vi "收集数据ICRA2024测试椭圆分裂.vi"() -> ()   [LabVIEW 2018]
doc: "Demonstrates the use of the Network Streams functions to send LED status to the myRIO target."
uses:
  <vilib>/ErrorRing/Error Ring.xnode
  <vilib>/vision/NI_Vision_Development_Module.lvlib
panel:
  out "面积":sgl[](array[numeric])
  out "面积":sgl
  out "数据总":dbl[][](array[numeric])
  out "i":i32[](array[numeric])
  out "aspect ratio":dbl[](array[numeric])
  out "D2":i32[](array[numeric])
  out "D1":i32[](array[numeric])
  out "field ratio":sgl[](array[numeric])
  out "field ratio":sgl=4.0
  out "时间":i32
  in  "打开数据记录":bool
  out "aspect ratio":dbl
  out "D2":i32
  out "D1":i32
  out "二值图":T1(plugin-control)
  in  "Search Rect (entire image)":T2={"Left"=200, "Top"=120, "Right"=2000, "Bottom"=1920, "Rotation"=0.0} {"Rotation" format="%.2f"; "Left" scale=0.0..1024.0; "Right" scale=0.0..1024.0}
  out "备用的椭圆角度":sgl
  in  "Number of Erosion":i32=10
  in  "椭圆磁场开关":bool=TRUE
  out "Image 7":T1(plugin-control)
  in  "Acquisition Control::Acquisition Frame Rate":dbl=19.50304412841797 min=1.4211589097976685 max=44.94382095336914
  out "Stopped":bool
  in  "Stop (F) 2":bool caption="Stop (F)"
  out "Objects 2":T3(array[cluster]) {"Aspect Ratio" format="%.2f"; "Orientation" format="%.2f"; "Area" format="%.2f"; "Object Center"."Y" format="%.2f"; "Object Center"."X" format="%.2f"}
  in  "Settings 2":T4={"Objects"=0, "Threshold"=128, "Reject Border"=FALSE, "Fill Holes"=FALSE, "Min Object Size"=TRUE, "Min Size"=20000, "Max Object Size"=FALSE, "Max Size"=100, "Show Search Area"=FALSE, "Show Center"=TRUE, "Show Bounding Box"=TRUE} {"Objects" items=["Bright Objects", "Dark Objects"]; "Threshold" min=1 max=999999999 step=1; "Max Size" min=1 max=999999999 step=1; "Min Size" min=1 max=999999999 step=1}
  in  "Range 2":cluster{"Lower value":sgl, "Upper value":sgl}={"Lower value"=0.0, "Upper value"=230.0} {"Upper value" format="%.2f"; "Lower value" format="%.2f"}
  in  "Pause":bool
  out "Array":dbl[](array[numeric])
  in  "Parameter Settings":T5(tab)=enum."Ribbon Oscillating Field" caption="Field Types"
  in  "fg":dbl
  in  "pg":dbl
  in  "dg":dbl
  in  "Ag":dbl
  in  "AoOF":dbl
  in  "fo":sgl
  in  "do":sgl
  in  "oo":sgl
  in  "po":sgl
  in  "cc":sgl
  in  "pc":sgl
  in  "wc":sgl
  in  "dc":sgl
  in  "Ac":dbl
  in  "pr":sgl
  in  "Ar":dbl=8.0
  in  "wr":sgl=18.0
  in  "dr":sgl
  in  "Dis phase step":dbl
  in  "Dis phase frequency (Hz)":dbl
  in  "Dis tumbling frequency (Hz)":dbl
  in  "Dis strength(mT)":dbl
  in  "Swa strength (mT)":dbl
  in  "Swa frequency (Hz)":dbl
  in  "Swa pitch angle (deg)":dbl
  in  "Swa direction angle (deg)":dbl
  in  "Swa ratio":dbl=1.0
  in  "Pitch Angle (rotating around Constant, deg)":dbl
  in  "Ratio (A/C)":sgl=4.0
  in  "Direction Angle (deg)":sgl
  in  "Pitch Angle (rotating around Origin, deg)":sgl
  in  "Frequency (Hz)":sgl=10.0
  in  "Strength (mT)":dbl=10.0
  in  "Ar 2":dbl=5.0 caption="Ar"
  in  "ratio":sgl=1.0
  in  "运动方向":sgl
  in  "长轴方向":sgl
  in  "wr  2":sgl=8.0
  in  "速度大小":sgl
  out "Numeric 5":i32
  in  "Stop":bool
  out "error out":errorcluster
  in  "Target IP Address":string="172.22.11.2"
  # "Overview: Magnetic field calculation, and send parameters to myRIO\nInstructions:\n1. Verify the value of Target IP Address. Set Visa resource name.\n2. Ensure RT Main.vi is already running. \n3. Run this VI. Set parameters of magnetic field."
  # "Strength (mT)"
  # "Pitch Angle (deg)"
  # "Direction Angle (deg)"
  # "Frequency (Hz)"
  # "Strength (mT)"
  # "Oscilation Frequency (Hz)"
  # "Oscilation Angle (deg)"
  # "Pitch Angle (deg)"
  # "Direction Angle (deg)"
  # "Strength (mT)"
  # "Frequency (Hz)"
  # "Pitch Angle (deg)"
  # "Direction Angle (deg)"
  # "Conical Angle (deg)"
  # "Strength (mT)"
  # "Frequency (Hz)"
  # "Pitch Angle (deg)"
  # "Direction Angle (deg)"
  # "Strength (mT)"
  # "Tumbling Frequency (Hz)"
  # "Phase Frequency (Hz)"
  # "Phase Step"
  # "Strength (mT)"
  # "Frequency (Hz)"
  # "Pitch Angle (deg)"
  # "Direction Angle (deg)"
  # "Ratio"
  # "Strength (mT)"
  # "Frequency (Hz)"
  # "Ratio (A/C)"
  # "Direction Angle (deg)"
  # "Pitch Angle (rotating around Origin, deg)"
  # "Pitch Angle (rotating around Constant, deg)"
  # "Strength (mT)"
  # "Frequency (Hz)"
  # "Pitch Angle  (deg)"
  # "longaxis"
  # "Direction Angle (deg)"
  # "ratio (l/s)"
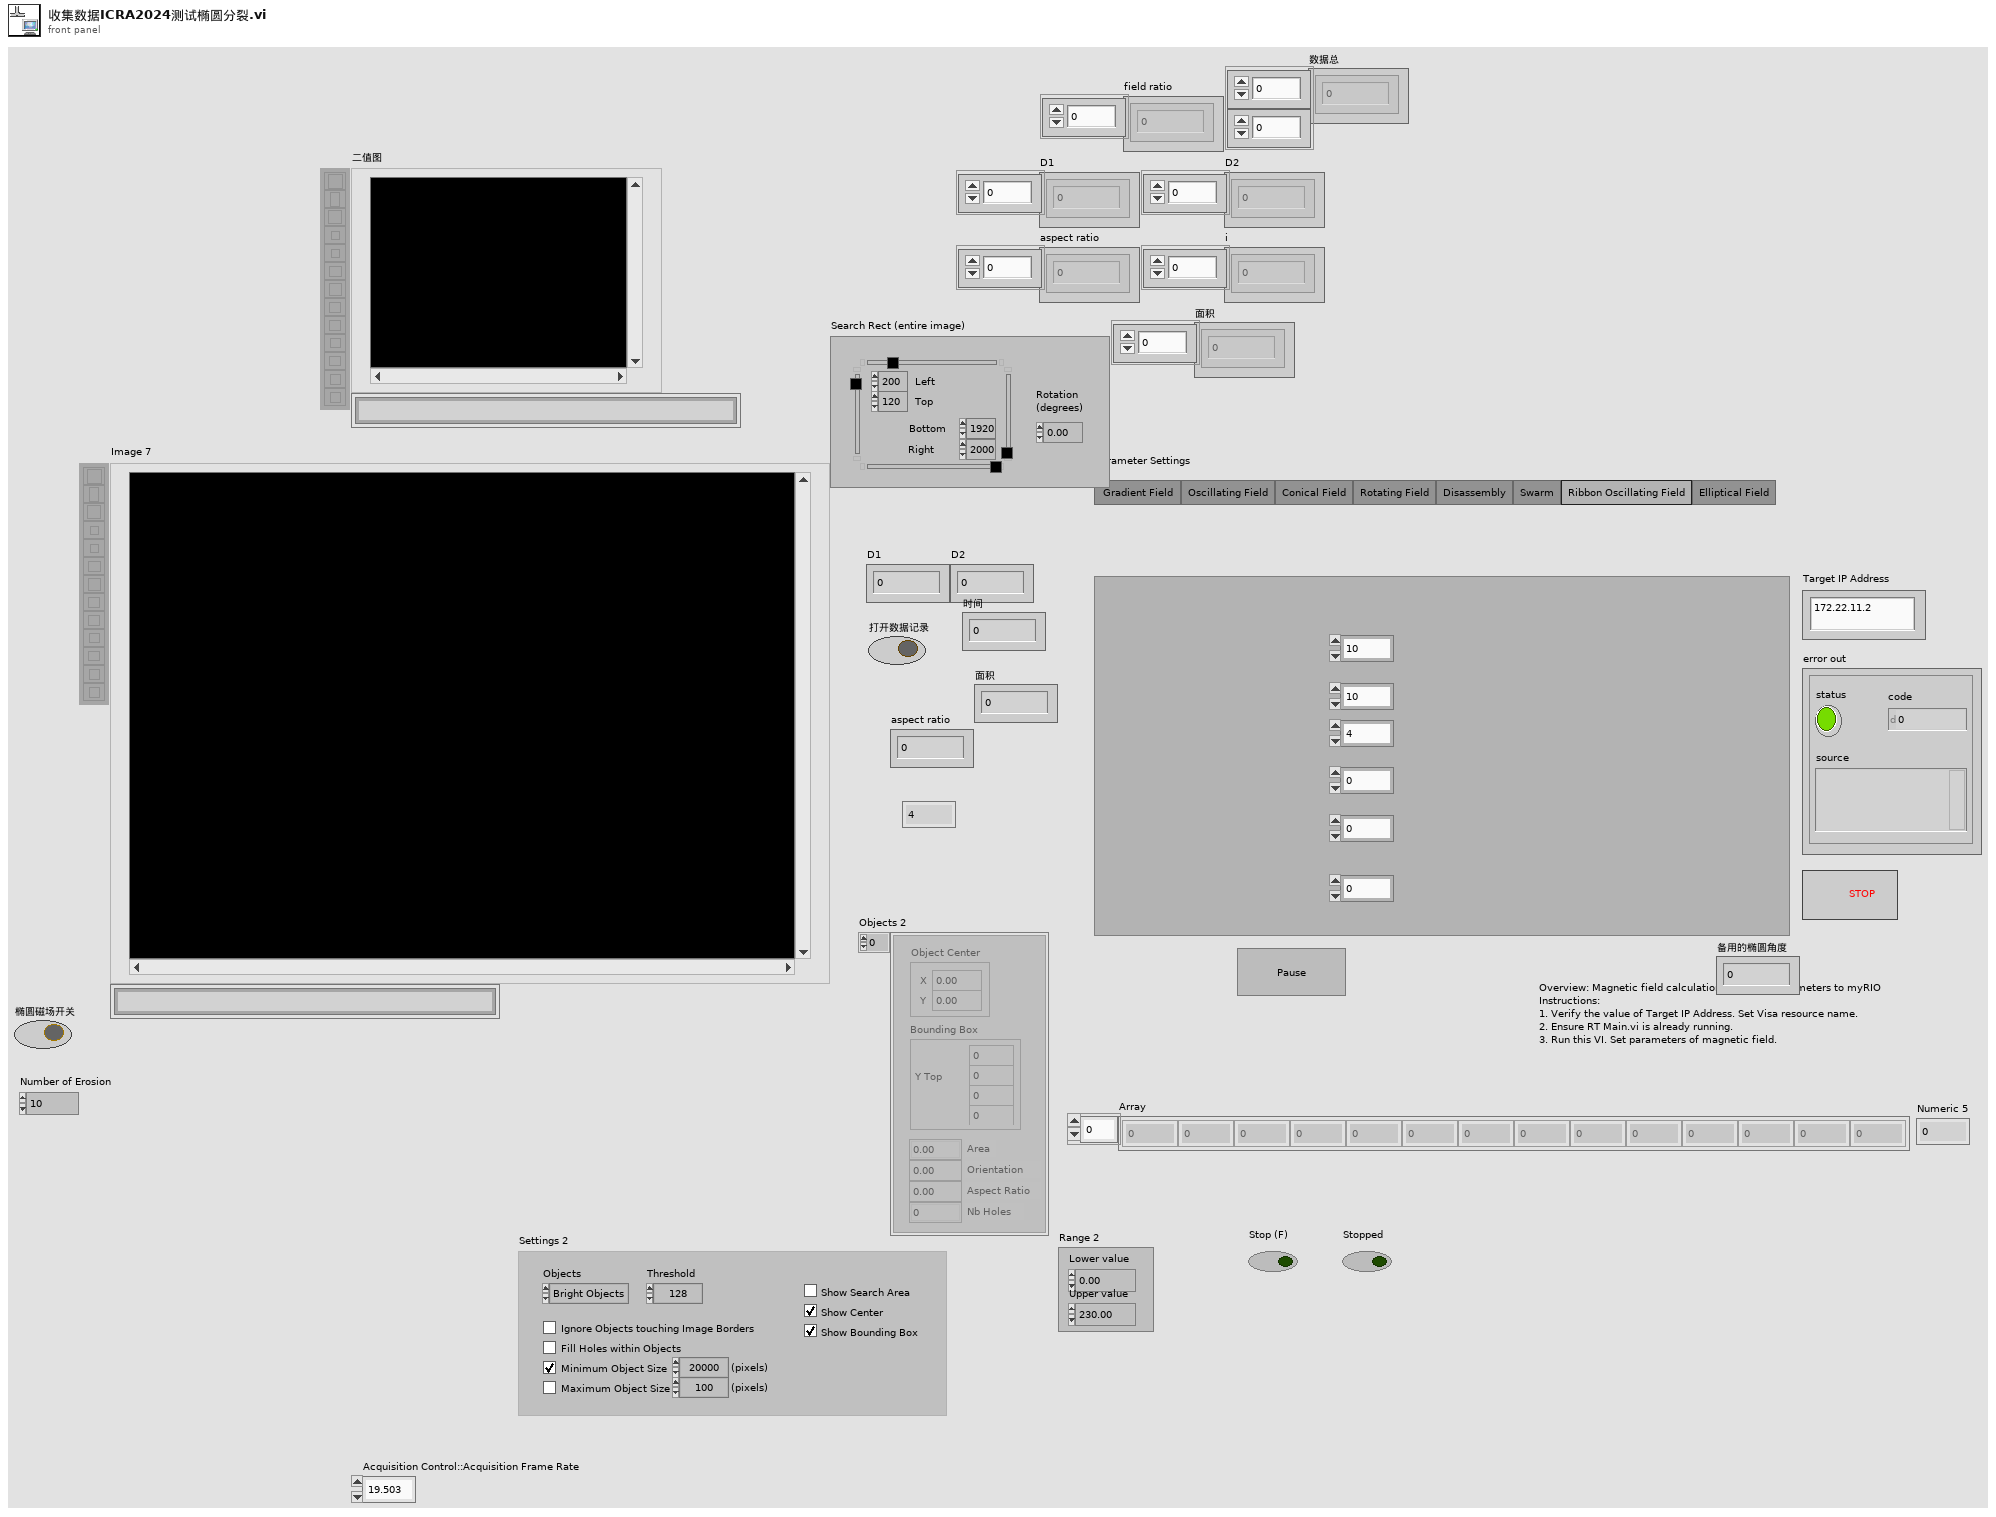
[diagram p1: front panel]
types:
  T1 = typedef "IMAQ Image.ctl" = refnum<image>
  T2 = typedef "IMAQ Rectangle" = cluster{"Left":i32, "Top":i32, "Right":i32, "Bottom":i32, "Rotation":dbl}
  T3 = cluster{"Object Center":cluster{"X":sgl, "Y":sgl}, "Bounding Box":cluster{"X Left":i32, "Y Top":i32, "X Right":i32, "Y Bottom":i32}, "Area":sgl, "Orientation":sgl, "Aspect Ratio":sgl, "Nb Holes":i32}[]
  T4 = cluster{"Objects":u16, "Threshold":i32, "Reject Border":bool, "Fill Holes":bool, "Min Object Size":bool, "Min Size":i32, "Max Object Size":bool, "Max Size":i32, "Show Search Area":bool, "Show Center":bool, "Show Bounding Box":bool}
  T5 = enum32{"Gradient Field ", "Oscillating Field", "Conical Field", "Rotating Field", "Disassembly", "Swarm", "Ribbon Oscillating Field", "Elliptical Field"}
  T6 = typedef "Image Type" = u32
  T7 = cluster{"Objects[0]":cluster{"Object Center":cluster{"X":sgl, "Y":sgl}, "Bounding Box":cluster{"X Left":i32, "Y Top":i32, "X Right":i32, "Y Bottom":i32}, "Area":sgl, "Orientation":sgl, "Aspect Ratio":sgl, "Nb Holes":i32}, "Objects[1]":cluster{"Object Center":cluster{"X":sgl, "Y":sgl}, "Bounding Box":cluster{"X Left":i32, "Y Top":i32, "X Right":i32, "Y Bottom":i32}, "Area":sgl, "Orientation":sgl, "Aspect Ratio":sgl, "Nb Holes":i32}, "Objects[2]":cluster{"Object Center":cluster{"X":sgl, "Y":sgl}, "Bounding Box":cluster{"X Left":i32, "Y Top":i32, "X Right":i32, "Y Bottom":i32}, "Area":sgl, "Orientation":sgl, "Aspect Ratio":sgl, "Nb Holes":i32}, "Objects[3]":cluster{"Object Center":cluster{"X":sgl, "Y":sgl}, "Bounding Box":cluster{"X Left":i32, "Y Top":i32, "X Right":i32, "Y Bottom":i32}, "Area":sgl, "Orientation":sgl, "Aspect Ratio":sgl, "Nb Holes":i32}, "Objects[4]":cluster{"Object Center":cluster{"X":sgl, "Y":sgl}, "Bounding Box":cluster{"X Left":i32, "Y Top":i32, "X Right":i32, "Y Bottom":i32}, "Area":sgl, "Orientation":sgl, "Aspect Ratio":sgl, "Nb Holes":i32}, "Objects[5]":cluster{"Object Center":cluster{"X":sgl, "Y":sgl}, "Bounding Box":cluster{"X Left":i32, "Y Top":i32, "X Right":i32, "Y Bottom":i32}, "Area":sgl, "Orientation":sgl, "Aspect Ratio":sgl, "Nb Holes":i32}, "Objects[6]":cluster{"Object Center":cluster{"X":sgl, "Y":sgl}, "Bounding Box":cluster{"X Left":i32, "Y Top":i32, "X Right":i32, "Y Bottom":i32}, "Area":sgl, "Orientation":sgl, "Aspect Ratio":sgl, "Nb Holes":i32}, "Objects[7]":cluster{"Object Center":cluster{"X":sgl, "Y":sgl}, "Bounding Box":cluster{"X Left":i32, "Y Top":i32, "X Right":i32, "Y Bottom":i32}, "Area":sgl, "Orientation":sgl, "Aspect Ratio":sgl, "Nb Holes":i32}, "Objects[8]":cluster{"Object Center":cluster{"X":sgl, "Y":sgl}, "Bounding Box":cluster{"X Left":i32, "Y Top":i32, "X Right":i32, "Y Bottom":i32}, "Area":sgl, "Orientation":sgl, "Aspect Ratio":sgl, "Nb Holes":i32}}
  T8 = cluster{"Object Center":cluster{"X":sgl, "Y":sgl}, "Bounding Box":cluster{"X Left":i32, "Y Top":i32, "X Right":i32, "Y Bottom":i32}, "Area":sgl, "Orientation":sgl, "Aspect Ratio":sgl, "Nb Holes":i32}
  T9 = cluster{"X Left":i32, "Y Top":i32, "X Right":i32, "Y Bottom":i32}
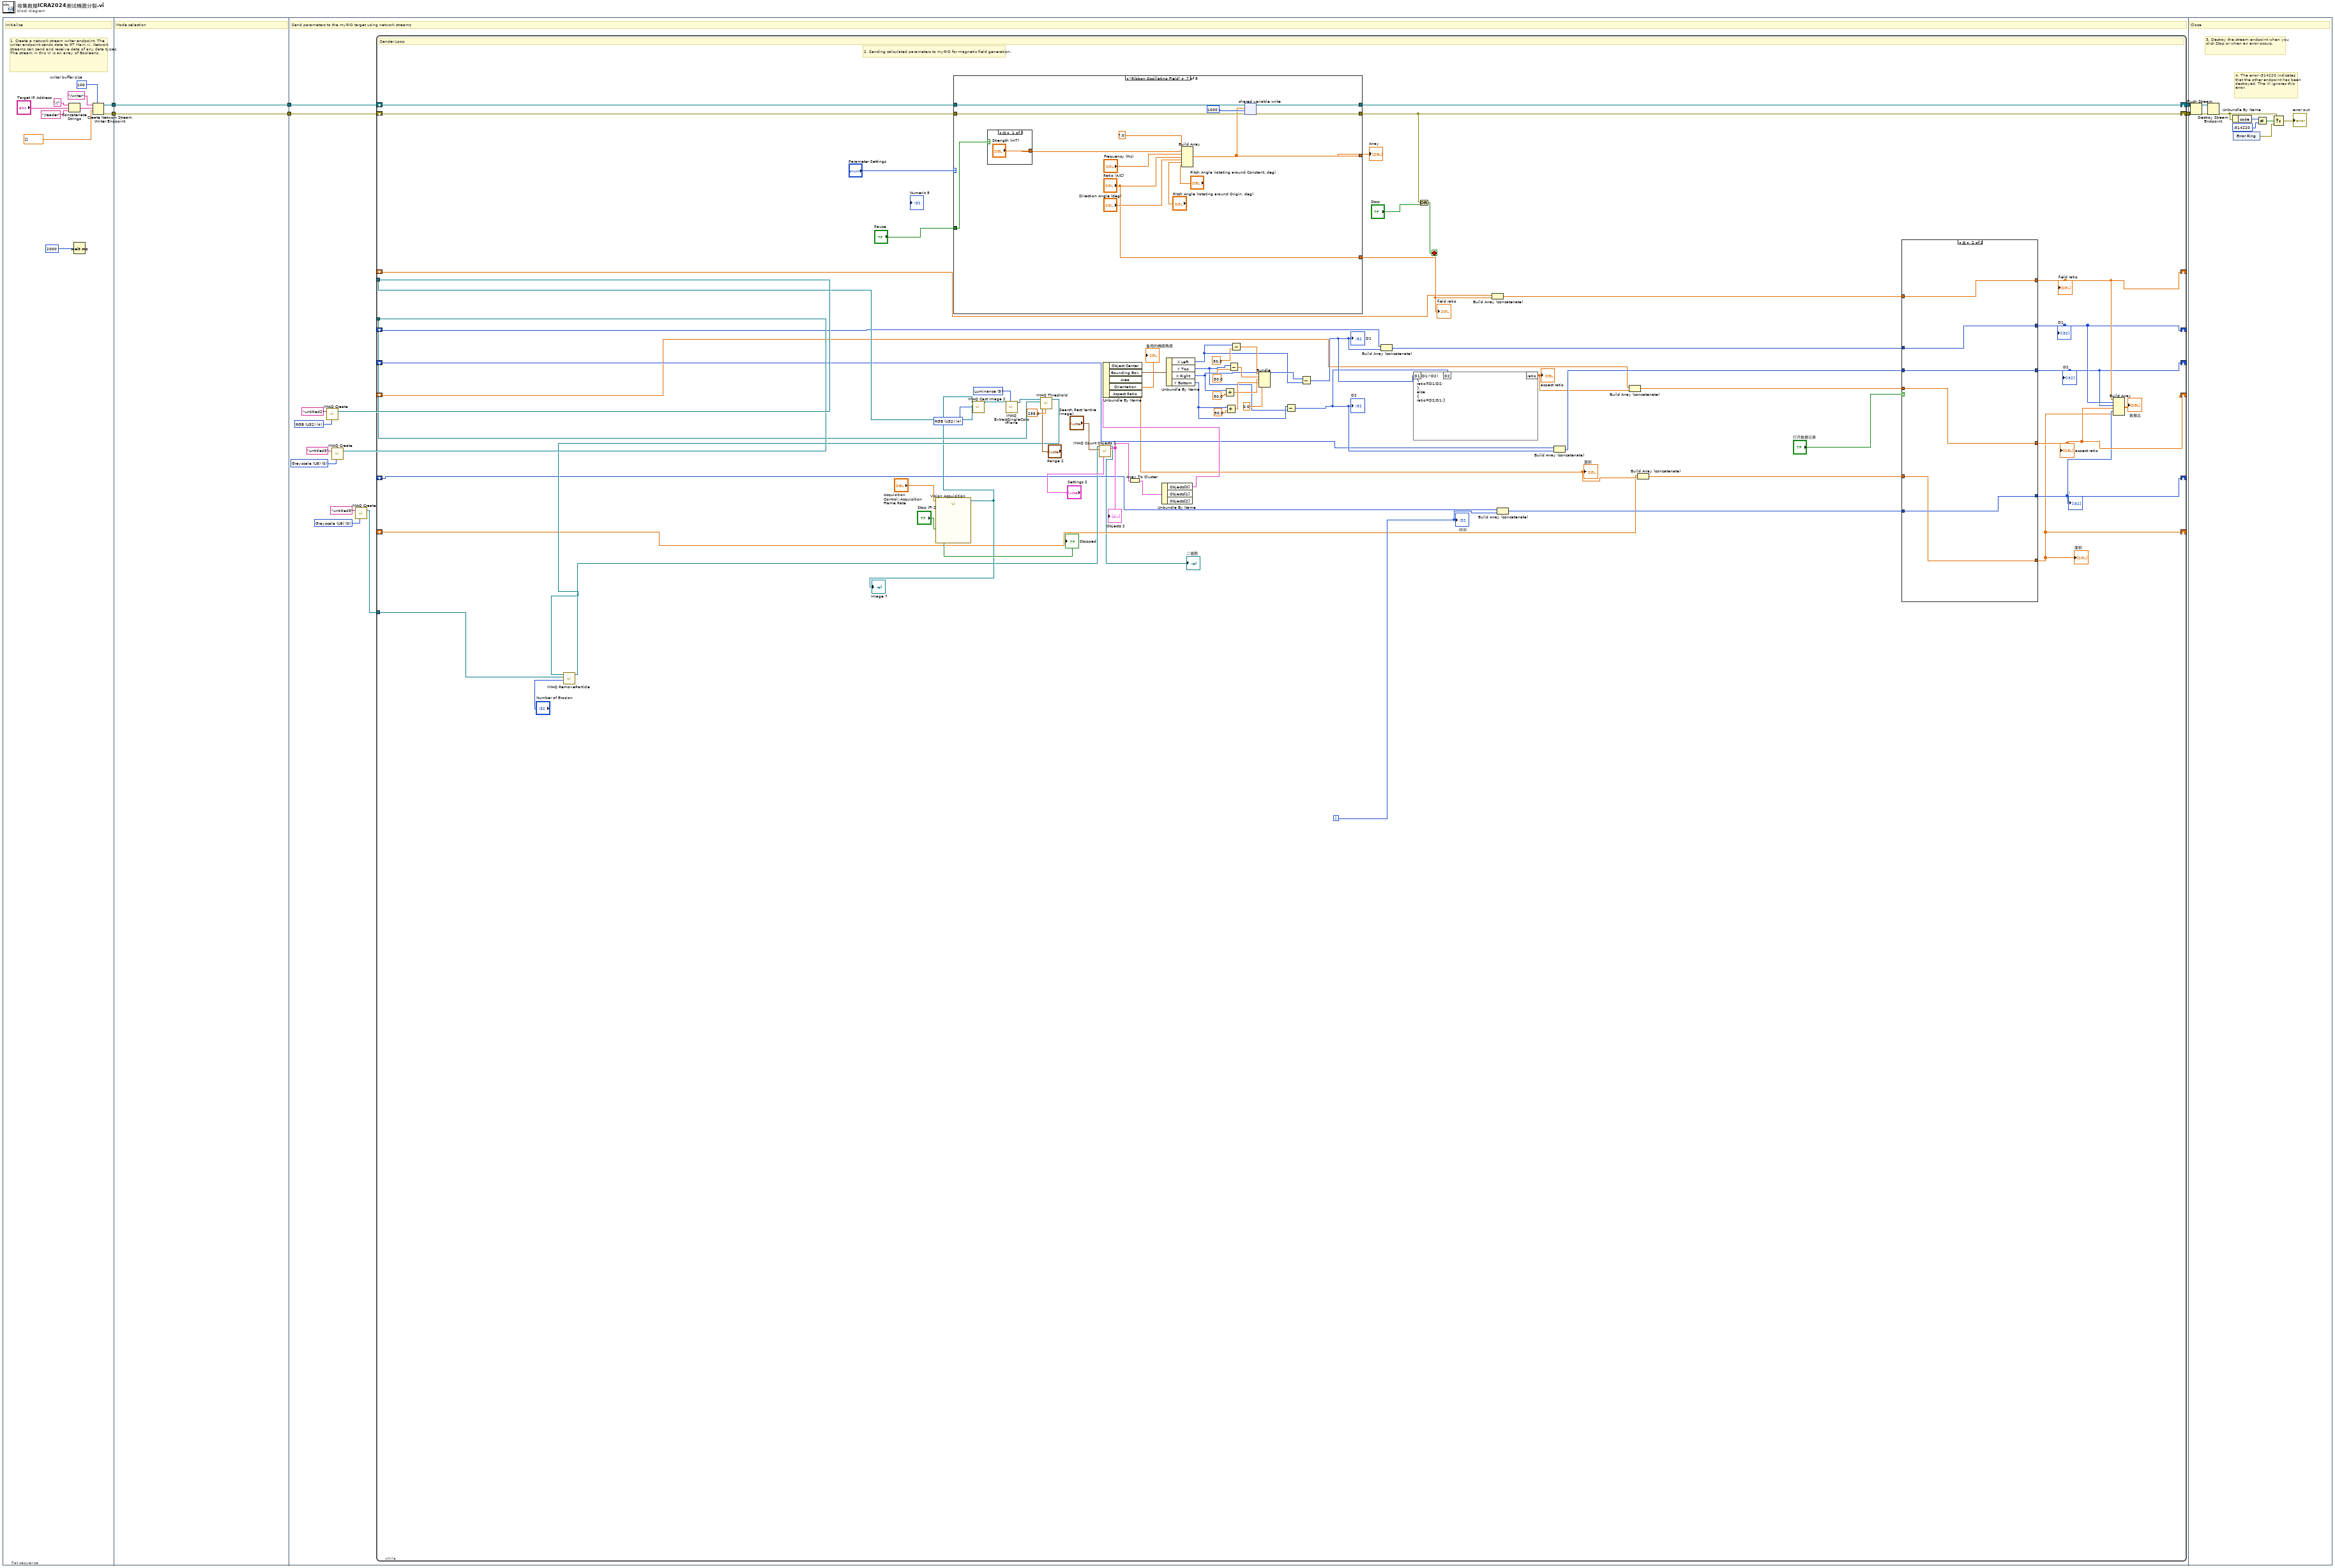
[diagram p0: block diagram]
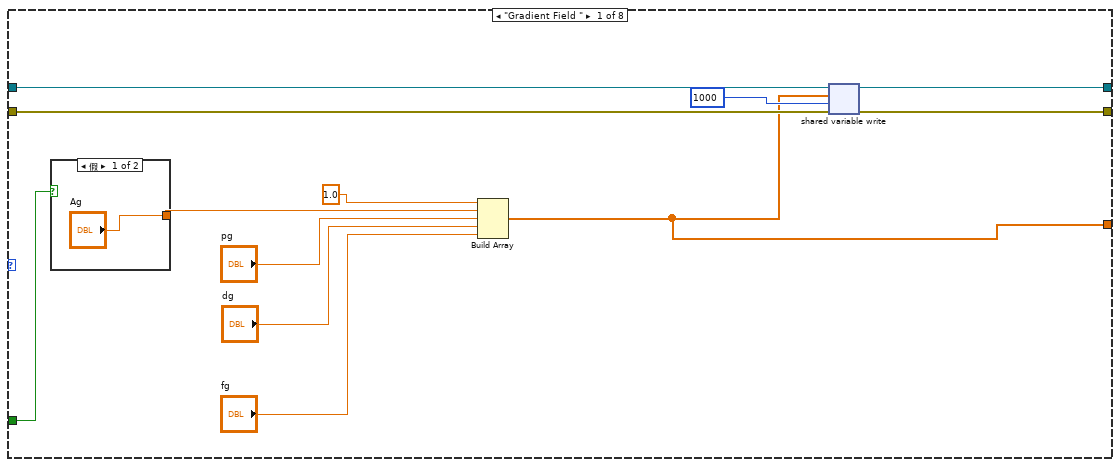
[diagram p3: hidden frame]
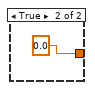
[diagram p4: hidden frame]
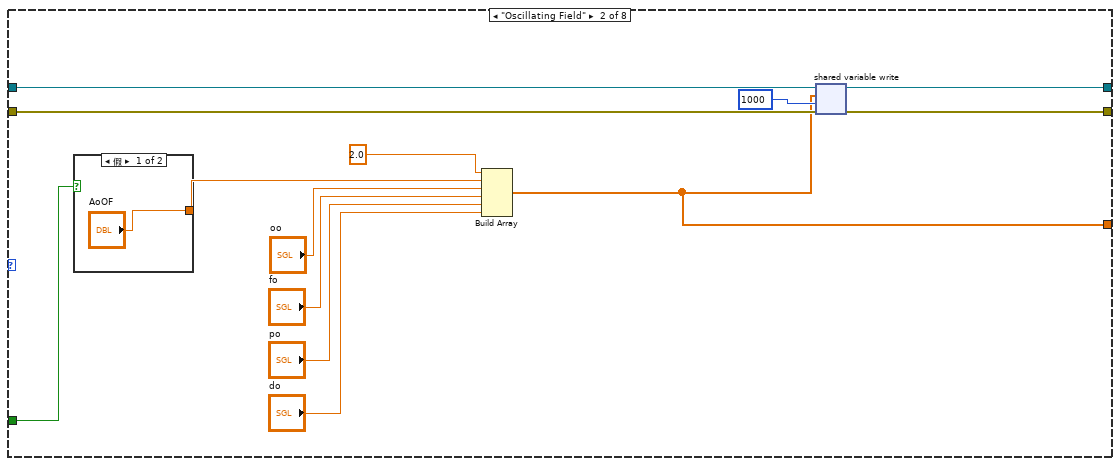
[diagram p5: hidden frame]
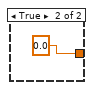
[diagram p6: hidden frame]
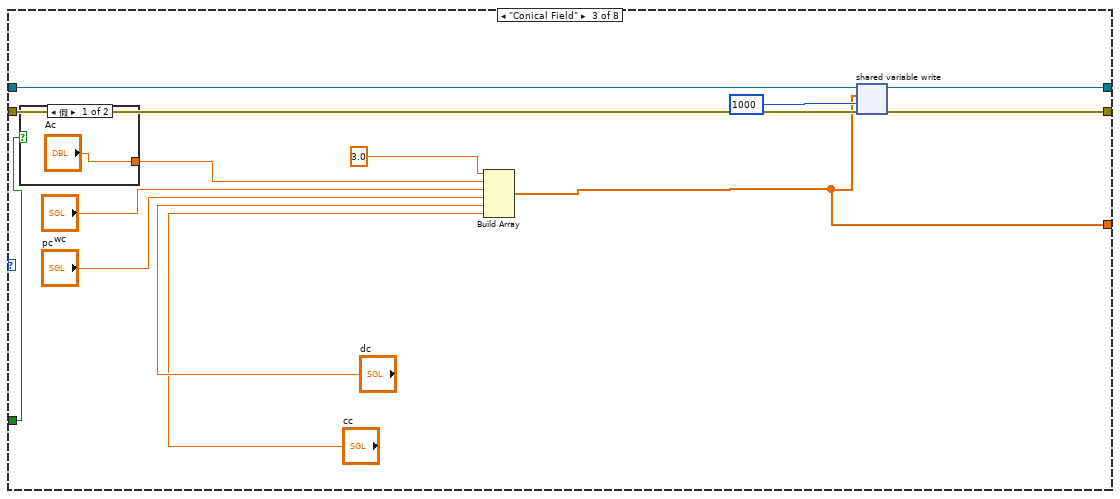
[diagram p7: hidden frame]
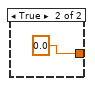
[diagram p8: hidden frame]
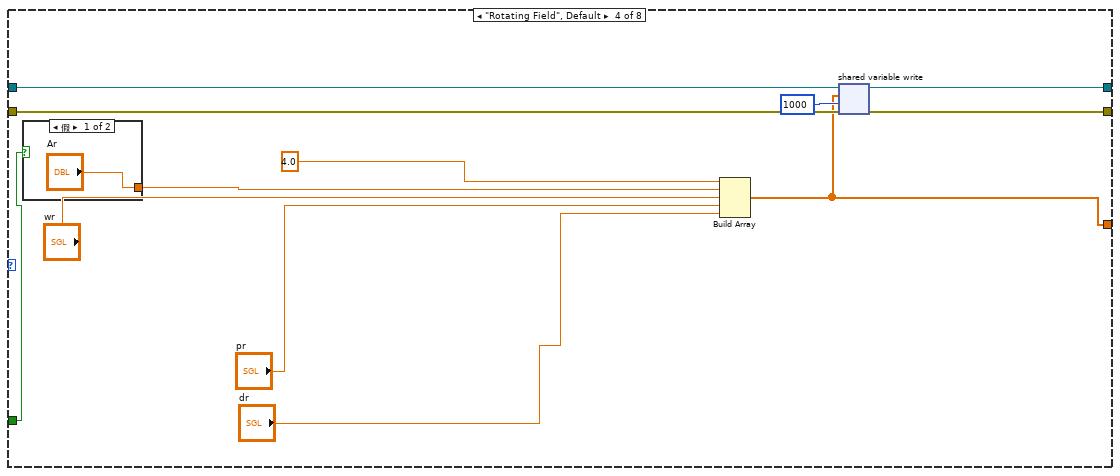
[diagram p9: hidden frame]
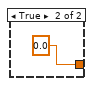
[diagram p10: hidden frame]
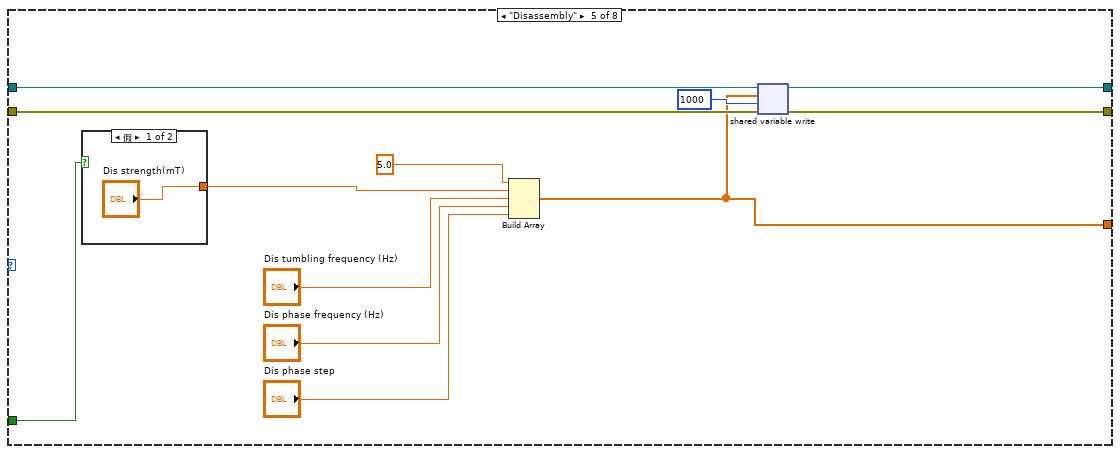
[diagram p11: hidden frame]
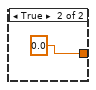
[diagram p12: hidden frame]
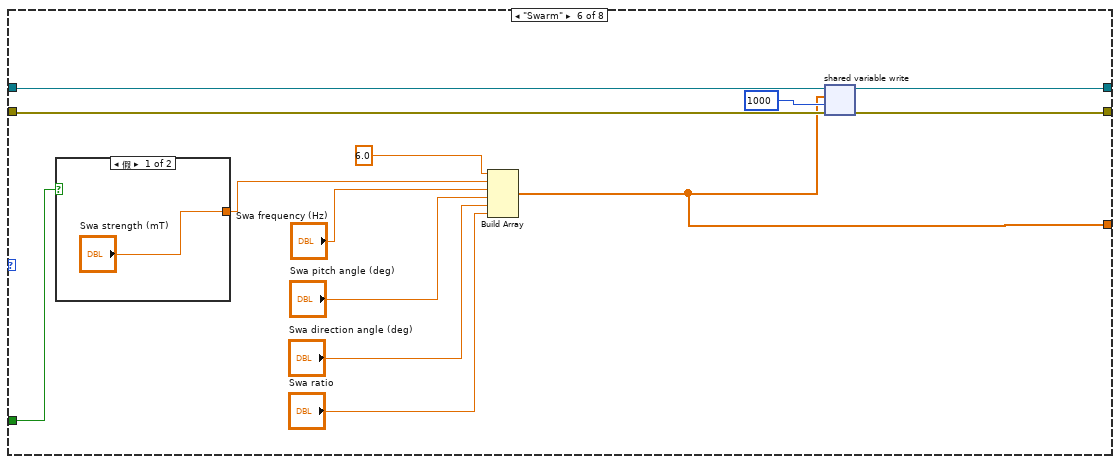
[diagram p13: hidden frame]
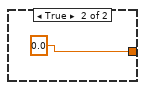
[diagram p14: hidden frame]
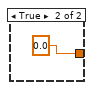
[diagram p15: hidden frame]
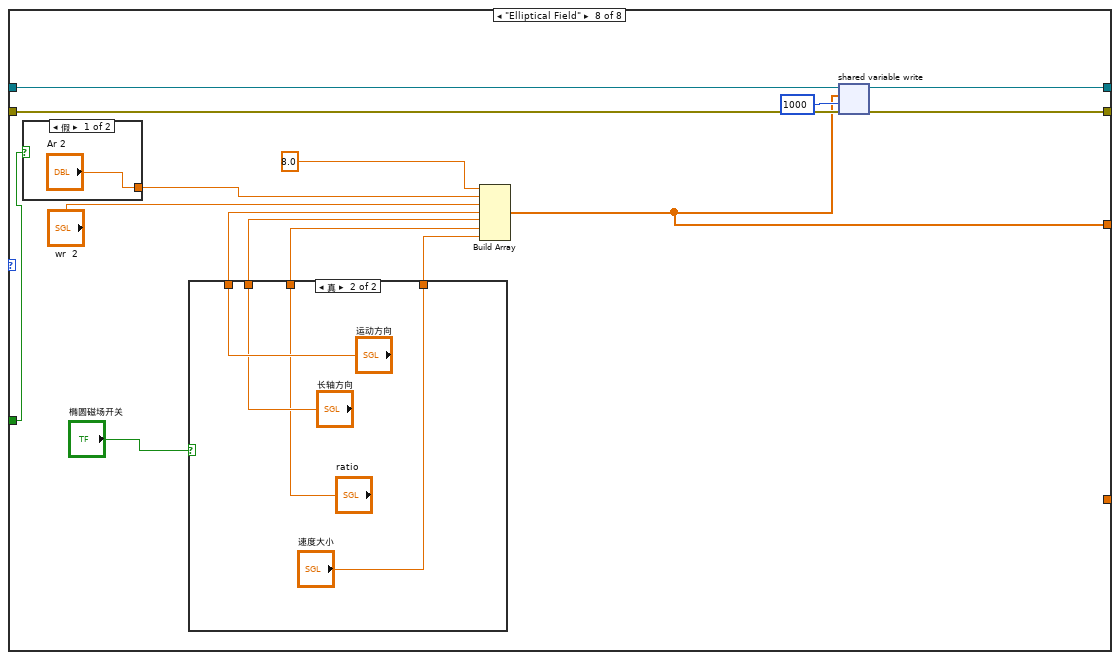
[diagram p16: hidden frame]
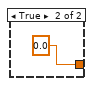
[diagram p18: hidden frame]
diagram:
  n1 = flat-sequence {
    tunnel: [w11] -> w2
    tunnel: [w10] -> w1
    tunnel: [w18] -> w4
    tunnel: [w17] -> w3
    tunnel: w1 -> [w17]
    tunnel: w2 -> [w18]
    tunnel: [w29] -> w6
    tunnel: w4 -> [w31]
    tunnel: [w28] -> w5
    tunnel: w3 -> [w30]
    tunnel: w6 -> [w243]
    tunnel: w5 -> [w240]
    frame #0 {
      w9 = 100  # writer buffer size
      # "1. Create a network stream writer endpoint. The writer endpoint sends data to RT Main.vi. Network streams can send and receive data of any data types. The stream in this VI is an array of Booleans."
      # "Initialize"
      n2 = Concatenate Strings("//", "Target IP Address", "/reader") -> (w16:string)
      n3 = Wait (ms)(milliseconds to wait=2000) -> ()  [unwired: 1 out]
      n4 = Create Network Stream Writer Endpoint(7:w9, 9:dbl[] [], 10:w16, 11:"/writer" ("reader name")) -> (0:w10:errorcluster, 3:w11:refnum<k21>)  [unwired: 3 in]
    }
    frame #1 {
      # "Mode selection"
    }
    frame #2 {
      w20 = T6 0 items=["Grayscale (U8)", "Grayscale (I16)", "Grayscale (SGL)", "Complex (CSG)", "RGB (U32)", "HSL (U32)", "RGB (U64)", "Grayscale (U16)"] ("Image Type")
      w24 = T6 0 items=["Grayscale (U8)", "Grayscale (I16)", "Grayscale (SGL)", "Complex (CSG)", "RGB (U32)", "HSL (U32)", "RGB (U64)", "Grayscale (U16)"] ("Image Type")
      w26 = T6 4 items=["Grayscale (U8)", "Grayscale (I16)", "Grayscale (SGL)", "Complex (CSG)", "RGB (U32)", "HSL (U32)", "RGB (U64)", "Grayscale (U16)"] ("Image Type")
      # "Send parameters to the myRIO target using network streams"
      n5 = call "IMAQ Create"("Image Name"="untitled2", "Image Type"=w26) -> ("New Image"=w23:T1)  [unwired: 3 in, 1 out]
      n6 = call "IMAQ Create"("Image Name"="untitled3", "Image Type"=w24) -> ("New Image"=w22:T1)  [unwired: 3 in, 1 out]
      n7 = call "IMAQ Create"("Image Name"="untitled3", "Image Type"=w20) -> ("New Image"=w19:T1)  [unwired: 3 in, 1 out]
      n8 = while {
        shift-right: [w99] -> w28
        shift-left: w30 -> [w101]
        shift-right: [w100] -> w29
        shift-left: w31 -> [w102]
        tunnel: w22 -> [w90]
        tunnel: w23 -> [w85]
        tunnel: w19 -> [w70]
        shift-right: [w42] -> _
        shift-left: _ -> [w55]
        shift-right: [w41] -> _
        shift-left: _ -> [w52]
        shift-right: [w40] -> _
        shift-left: _ -> [w49]
        shift-right: [w39] -> _
        shift-left: _ -> [w46]
        shift-right: [w38] -> _
        shift-left: _ -> [w43]
        shift-right: [w34] -> _
        shift-left: _ -> [w33]
        i -> [w45]
        stop <- w89 stop-if-true
        w84 = T6 4 items=["Grayscale (U8)", "Grayscale (I16)", "Grayscale (SGL)", "Complex (CSG)", "RGB (U32)", "HSL (U32)", "RGB (U64)", "Grayscale (U16)"] ("Image Type")
        w95 = 5 items=["Red", "Green", "Blue", "Hue", "Saturation", "Luminance", "Value", "Intensity"] ("Color Plane")
        # "2. Sending calculated parameters to myRIO for magnetic field generation."
        # "Sender Loop"
        n9 = call "Vision Acquisition"("Acquisition Control::Acquisition Frame Rate"="Acquisition Control::Acquisition Frame Rate", "Stop (F)"="Stop (F) 2") -> ("Image Out"=w62:T1, "Stopped"=→"Stopped":bool)  [unwired: 23 in, 1 out]
        "Image 7" <- w62
        n10 = case shown="\"Ribbon Oscillating Field\"" "Parameter Settings" {
          tunnel: w102 -> [w120 w135 w150 w164 w178 w192 w210 w226]
          tunnel: w101 -> [w117 w134 w149 w163 w176 w191 w208 w225]
          tunnel: [w119 w133 w147 w162 w177 w190 w209 w224] -> w100
          tunnel: [w118 w132 w148 w161 w175 w189 w207 w223] -> w99
          tunnel: [w113 w126 w141 w156 w169 w184 w205 w218] -> w98
          tunnel: "Pause" -> [w111 w124 w139 w154 w168 w183 w201 w216]
          tunnel: [_ _ _ _ _ _ "Ratio (A/C)" _] -> w57
          frame "Gradient Field " {
            n11 = case shown="假" w111 {
              tunnel: ["Ag" 0.0] -> w112
              frame False {
              }
              frame True {
              }
            }
            n12 = Build Array(1.0, w112, "pg", "dg", "fg") -> (w113:dbl[])
            n13 = shared-variable-write(w120, w117, w113, 1000 ("timeout ms (-1)")) -> (w119:refnum<k21>, w118:errorcluster)  [unwired: 1 out]
          }
          frame "Oscillating Field" {
            n14 = case shown="假" w124 {
              tunnel: ["AoOF" 0.0] -> w125
              frame False {
              }
              frame True {
              }
            }
            n15 = Build Array(2.0, w125, "oo", "fo", "po", "do") -> (w126:dbl[])
            n16 = shared-variable-write(w135, w134, w126, 1000 ("timeout ms (-1)")) -> (w133:refnum<k21>, w132:errorcluster)  [unwired: 1 out]
          }
          frame "Conical Field" {
            # "FG"
            n17 = case shown="假" w139 {
              tunnel: ["Ac" 0.0] -> w140
              frame False {
              }
              frame True {
              }
            }
            n18 = Build Array(3.0, w140, "wc", "pc", "dc", "cc") -> (w141:dbl[])
            n19 = shared-variable-write(w150, w149, w141, 1000 ("timeout ms (-1)")) -> (w147:refnum<k21>, w148:errorcluster)  [unwired: 1 out]
          }
          frame "Rotating Field", Default {
            n20 = case shown="假" w154 {
              tunnel: ["Ar" 0.0] -> w155
              frame False {
              }
              frame True {
              }
            }
            n21 = Build Array(4.0, w155, "wr", "pr", "dr") -> (w156:dbl[])
            n22 = shared-variable-write(w164, w163, w156, 1000 ("timeout ms (-1)")) -> (w162:refnum<k21>, w161:errorcluster)  [unwired: 1 out]
          }
          frame "Disassembly" {
            n23 = case shown="假" w168 {
              tunnel: ["Dis strength(mT)" 0.0] -> w173
              frame False {
              }
              frame True {
              }
            }
            n24 = Build Array(5.0, w173, "Dis tumbling frequency (Hz)", "Dis phase frequency (Hz)", "Dis phase step") -> (w169:dbl[])
            n25 = shared-variable-write(w178, w176, w169, 1000 ("timeout ms (-1)")) -> (w177:refnum<k21>, w175:errorcluster)  [unwired: 1 out]
          }
          frame "Swarm" {
            n26 = case shown="假" w183 {
              tunnel: ["Swa strength (mT)" 0.0] -> w182
              frame False {
              }
              frame True {
              }
            }
            n27 = Build Array(6.0, w182, "Swa frequency (Hz)", "Swa pitch angle (deg)", "Swa direction angle (deg)", "Swa ratio") -> (w184:dbl[])
            n28 = shared-variable-write(w192, w191, w184, 1000 ("timeout ms (-1)")) -> (w190:refnum<k21>, w189:errorcluster)  [unwired: 1 out]
          }
          frame "Ribbon Oscillating Field" {
            n29 = case shown="假" w201 {
              tunnel: ["Strength (mT)" 0.0] -> w200
              frame False {
              }
              frame True {
              }
            }
            n30 = Build Array(7.0, w200, "Frequency (Hz)", "Ratio (A/C)", "Direction Angle (deg)", "Pitch Angle (rotating around Origin, deg)", "Pitch Angle (rotating around Constant, deg)") -> (w205:dbl[])
            n31 = shared-variable-write(w210, w208, w205, 1000 ("timeout ms (-1)")) -> (w209:refnum<k21>, w207:errorcluster)  [unwired: 1 out]
          }
          frame "Elliptical Field" {
            n32 = case shown="假" w216 {
              tunnel: ["Ar 2" 0.0] -> w217
              frame False {
              }
              frame True {
              }
            }
            n33 = case shown="真" "椭圆磁场开关" {
              tunnel: [_ "运动方向"] -> w221
              tunnel: [_ "长轴方向"] -> w220
              tunnel: [_ "ratio"] -> w215
              tunnel: [_ "速度大小"] -> w214
              frame False {
              }
              frame True {
              }
            }
            n34 = Build Array(8.0, w217, "wr  2", w221, w220, w215, w214) -> (w218:dbl[])
            n35 = shared-variable-write(w226, w225, w218, 1000 ("timeout ms (-1)")) -> (w224:refnum<k21>, w223:errorcluster)  [unwired: 1 out]
          }
        }
        "Array" <- w98
        "field ratio" <- w57
        n36 = call "IMAQ Cast Image 2"("Image Src"=w62, "Image Dst"=w85, "Image Type"=w84) -> ("Image Dst Out"=w86:T1)  [unwired: 11 in, 1 out]
        n37 = call "IMAQ ExtractSingleColorPlane"("Color Plane"=w95, "Image Src"=w86) -> ("Image Dst Out"=w68:T1)  [unwired: 8 in, 1 out]
        n38 = call "IMAQ Threshold"("Replace Value"=sgl 255.0, "Range"="Range 2", "Image Dst"=w90, "Image Src"=w68) -> ("Image Dst Out"=w71:T1)  [unwired: 6 in, 1 out]
        n39 = call "IMAQ RemoveParticle"("Number of Erosion"="Number of Erosion", "Image Dst"=w70, "Image Src"=w71) -> ("Image Dst Out"=w61:T1)  [unwired: 7 in, 1 out]
        n40 = call "IMAQ Count Objects 2"("Settings"="Settings 2", "Search Rect (entire image)"="Search Rect (entire image)", "Image"=w61) -> ("Image Out"=→"二值图":T1, "Objects"=w91:T3)  [unwired: 4 in, 3 out]
        "Objects 2" <- w91
        n41 = Array To Cluster(array=w91) -> (cluster=w73:T7)
        n42 = Unbundle By Name(w73) -> ("Objects[0]"=w72:T8)  [unwired: 2 out]
        n43 = Unbundle By Name(w72) -> ("Bounding Box"=w83:T9, "Area"=w36:sgl, "Orientation"=→"备用的椭圆角度":sgl)  [unwired: 2 out]
        "面积" <- w36
        n44 = Unbundle By Name(w83) -> ("X Left"=w64:i32, "Y Top"=w59:i32, "X Right"=w65:i32, "Y Bottom"=w60:i32)
        n45 = Add(x=w65, y=50.0) -> (x+y=w76:dbl)
        n46 = Add(x=w60, y=50.0) -> (x+y=w75:dbl)
        n47 = Subtract(x=w59, y=50.0) -> (x-y=w77:dbl)
        n48 = Subtract(x=w64, y=50.0) -> (x-y=w78:dbl)
        n49 = Bundle(w78, w77, w76, w75, 0.0) -> ()  [unwired: 1 in, 1 out]
        n50 = Subtract(x=w60, y=w59) -> (x-y=w51:i32)
        "D2" <- w51
        n51 = Subtract(x=w65, y=w64) -> (x-y=w54:i32)
        "D1" <- w54
        n52 = Build Array (concatenate)(w52, w54) -> (w53:i32[])
        n53 = formula code="if (D1>D2)\n{\nratio=D1/D2;\n}\nelse\n{\nratio=D2/D1;}"("D1"=w54, "D2"=w51) -> ("ratio"=w48:dbl)
        "aspect ratio" <- w48
        n54 = Or(x=w99, y="Stop") -> (x .or. y?=w89:bool)
        n55 = Build Array (concatenate)(w55, w57) -> (w56:sgl[])
        n56 = Build Array (concatenate)(w43, w45) -> (w44:i32[])
        n57 = Build Array (concatenate)(w49, w51) -> (w50:i32[])
        n58 = Build Array (concatenate)(w46, w48) -> (w47:dbl[])
        n59 = Build Array (concatenate)(w33, w36) -> (w35:sgl[])
        n60 = case shown="真" "打开数据记录" {
          tunnel: [_ w109] -> w42
          tunnel: w56 -> [_ w109]
          tunnel: [_ w108] -> w41
          tunnel: w53 -> [_ w108]
          tunnel: [_ w107] -> w40
          tunnel: w50 -> [_ w107]
          tunnel: [_ w106] -> w39
          tunnel: w47 -> [_ w106]
          tunnel: [_ w105] -> w38
          tunnel: w44 -> [_ w105]
          tunnel: [_ w104] -> w34
          tunnel: w35 -> [_ w104]
          frame False {
          }
          frame True {
          }
        }
        "field ratio" <- w42
        "D1" <- w41
        "D2" <- w40
        "aspect ratio" <- w39
        "i" <- w38
        "面积" <- w34
        n61 = Build Array(w42, w41, w40, w39, w38, w34) -> (→"数据总":dbl[][])
        "时间" <- w45
      }
    }
    frame #3 {
      # "4. The error -314220 indicates that the other endpoint has been destroyed. The VI ignores this error."
      # "3. Destroy the stream endpoint when you click Stop or when an error occurs."
      # "Close"
      n62 = Flush Stream(8:w240, 11:w243) -> (0:w241:errorcluster, 3:w242:refnum<k21>)  [unwired: 2 in, 1 out]
      n63 = Destroy Stream Endpoint(8:w241, 11:w242) -> (0:w235:errorcluster)
      n64 = Unbundle By Name(w235) -> ("code"=w239:i32)
      n65 = xnode "Error Ring"() -> ("错误输出"=w236:errorcluster)
      n66 = Not Equal?(x=w239, y=-314220) -> (x != y?=w237:bool)
      n67 = Select(t=w235, s=w237, f=w236) -> (s? t:f=→"error out":errorcluster)
    }
  }
